vi "F Distribution.vi"(2 "m":i32=1 format="%0.0f", 3 "n":i32=1 format="%0.0f", 4 "x":dbl format="%0.4f") -> (0 "error":i32, 1 "probability":dbl format="%0.4f")   [LabVIEW 2017, in "NI_AALPro.lvlib"]
doc: "LabVIEW no longer supports this VI. Use the Continuous CDF VI (F instance) instead. Computes the one-sided <B>probability</B>, p, of the F-distributed random variable, F, with the specified <B>n</B> and <B>m</B> degrees of freedom. The F Distribution VI computes the one-sided <B>probability</B> such that the following condition is satisfied: p = Prob{F[<B>n</B>, <B>m</B>] <= <B>x</B>}, where F is F-distributed, p is the <B>probability</B>, <B>n</B> specifies the first degree of freedom, <B>m</B> specifies the second degree of freedom, and <B>x</B> is the value."
uses:
  <vilib>/Analysis/NI_AALPro.lvlib
  <resource>/lvanlys.dll
panel:
  # "F Distribution"
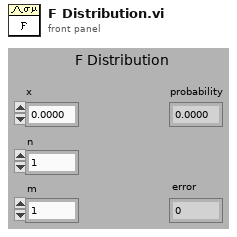
[diagram p1: front panel]
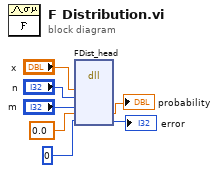
[diagram p0: block diagram]
diagram:
  n1 = dll-call lib="e:/builds/penguin/labview/branches/2017/dev/dist/resource/lvanlys.*" fn="FDist_head"("x"="x", "n"="n", "m"="m", 0.0, 0) -> (→"probability":dbl, →"error":i32)  [unwired: 7 in, 2 out]
